vi "TestVirtual1.vi"(0 "reference in":refnum<class "G#BaseClass1_IG#BaseInterface.lvclass">, 5 "error in (no error)":errorcluster) -> (14 "reference out":refnum<class "G#BaseClass1_IG#BaseInterface.lvclass">, 15 "MethodName":string[](array[string]), 19 "error out":errorcluster)   [LabVIEW 2010, in "G#BaseClass1_IG#BaseInterface.lvclass"]
uses:
  G#BaseClass1_IG#BaseInterface.lvclass
  G#BaseClass1.lvclass
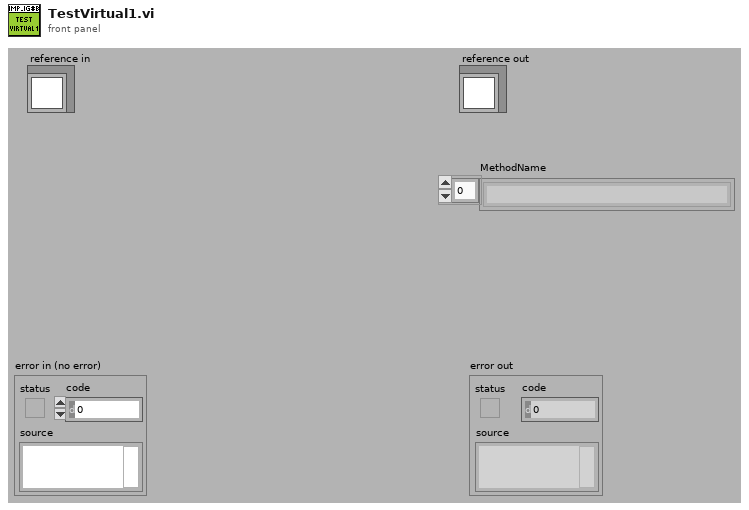
[diagram p1: front panel]
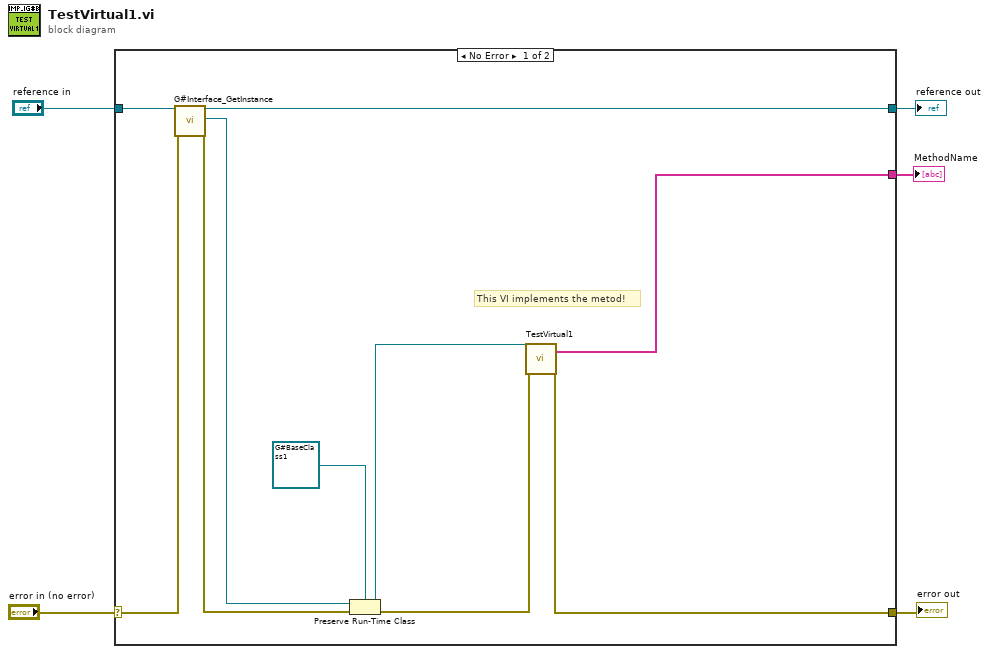
[diagram p0: block diagram]
diagram:
  n1 = case shown="No Error" "error in (no error)" {
    selector: "error in (no error)" -> [w13 w17]
    tunnel: [w10 w17] -> w4
    tunnel: [w14 w16] -> w2
    tunnel: "reference in" -> [w15 w16]
    tunnel: [w6 _] -> w1
    frame No Error {
      # "This VI implements the metod!"
      n2 = call-dynamic "G#Interface_GetInstance.vi"("reference in"=w15, "error in (no error)"=w13) -> ("reference out"=w14:refnum<class "G#BaseClass1_IG#BaseInterface.lvclass">, "G#Object"=w9:refnum<class "G#Object.lvclass">, "error out"=w12:errorcluster)  [unwired: 14 in, 1 out]
      n3 = Preserve Run-Time Class(object in=w9, error in=w12, 2:refnum<class "G#BaseClass1.lvclass"> refnum ("reference in")) -> (object out=w7:refnum<class "G#BaseClass1.lvclass">, error out=w11:errorcluster)
      n4 = call-dynamic "TestVirtual1.vi"("reference in"=w7, "error in (no error)"=w11) -> ("MethodName"=w6:string[], "error out"=w10:errorcluster)  [unwired: 15 in, 1 out]
    }
    frame Error {
    }
  }
  "error out" <- w4
  "reference out" <- w2
  "MethodName" <- w1
